vi "Write Logger.vi"(10 "Logger":T1={"Log Directory"=path "", "Log Filename Base"="", "Max records per file"=1000, "Comment"=""} {"Max records per file" min=100 max=1000000}, 11 "Logger in":refnum<class "Log.lvclass">) -> (3 "Logger out":refnum<class "Log.lvclass">)   [LabVIEW 2013, in "Log.lvclass"]
uses:
  Log.lvclass
  Configuration/Log.ctl
  Log.lvclass/Log.ctl
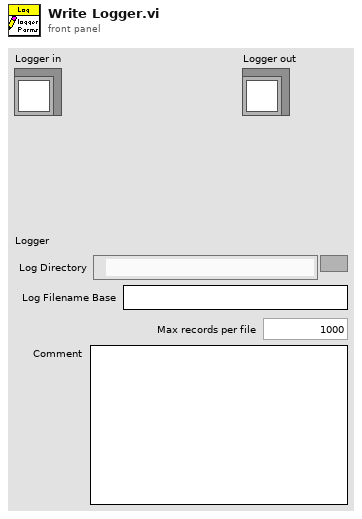
[diagram p1: front panel]
types:
  T1 = typedef "Log.ctl" = cluster{"Log Directory":path, "Log Filename Base":string, "Max records per file":u32, "Comment":string}
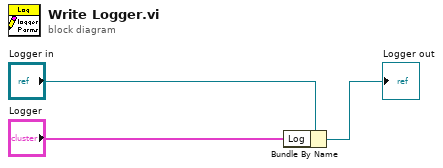
[diagram p0: block diagram]
diagram:
  n1 = Bundle By Name(cluster="Logger in", "Log"="Logger") -> (→"Logger out":refnum<class "Log.lvclass">)
